vi "main.vi"(11 "VI Refnum":refnum<vi>) -> ()   [LabVIEW 2013]
panel:
  out "Array":string[](array[string])
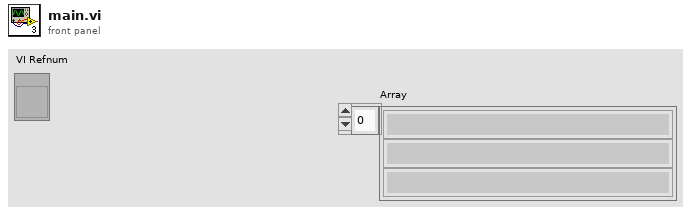
[diagram p1: front panel]
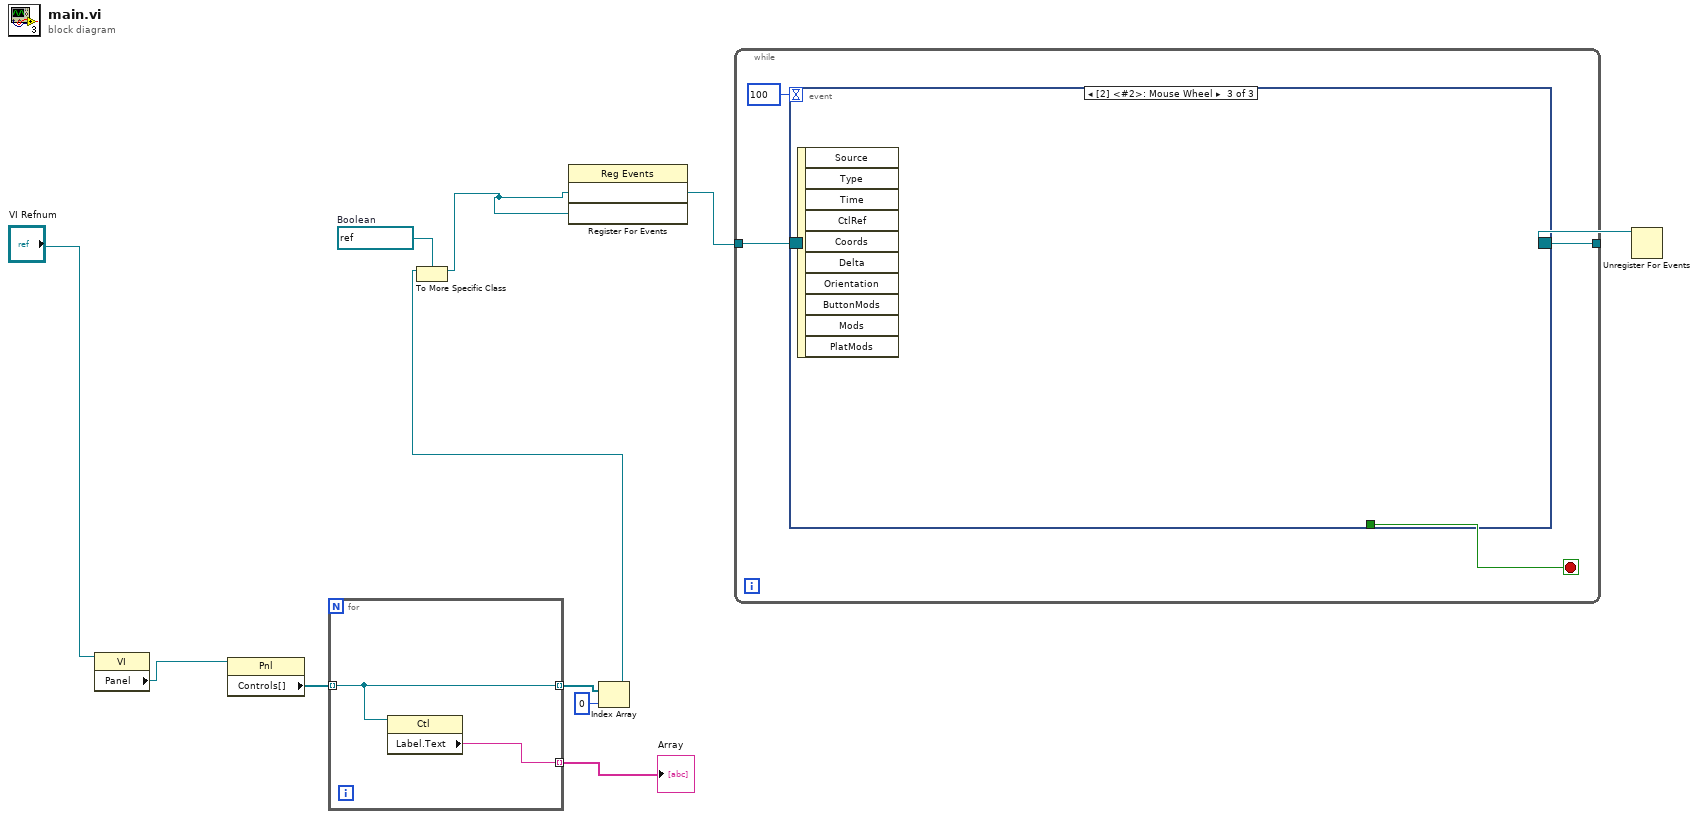
[diagram p0: block diagram]
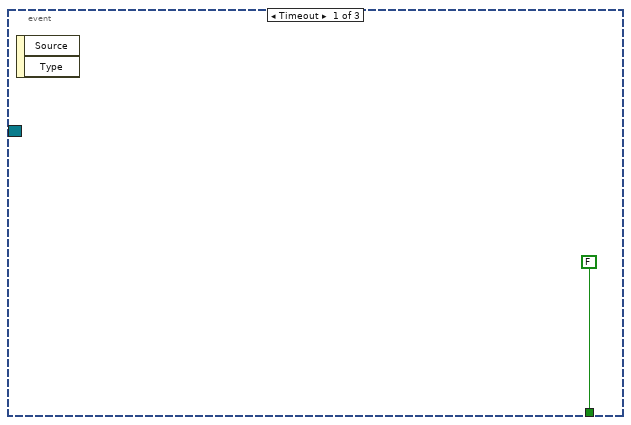
[diagram p2: hidden frame]
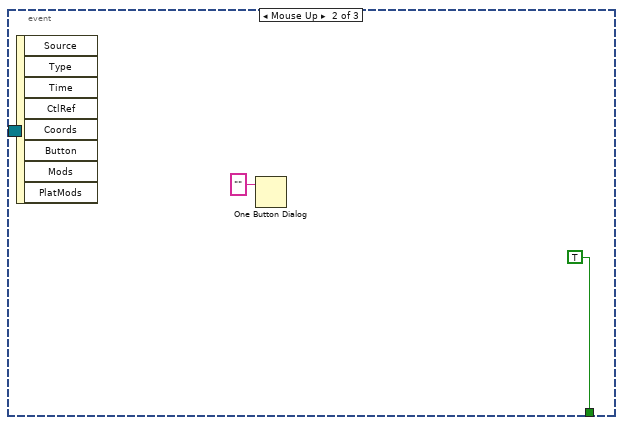
[diagram p3: hidden frame]
diagram:
  w2 = refnum<vi> refnum  # Boolean
  n1 = property class="VI"(reference="VI Refnum") -> ("Panel"=w10:refnum<vi>)  [unwired: 1 in, 2 out]
  n2 = property class="Pnl"(reference=w10) -> ("Controls[]"=w9:refnum<vi>[])  [unwired: 1 in, 2 out]
  n3 = for {
    tunnel: w9 -> [w12] mode=indexing
    tunnel: [w13] -> w8 mode=indexing
    tunnel: [w12] -> w6 mode=indexing
    n4 = property class="Ctl"(reference=w12) -> ("Label.Text"=w13:string)  [unwired: 1 in, 2 out]
  }
  "Array" <- w8
  n5 = Index Array(array=w6, index=0) -> (element=w1:refnum<vi>)
  n6 = To More Specific Class(target class=w2, reference=w1) -> (specific class reference=w3:refnum<vi>)  [unwired: 1 in, 1 out]
  n7 = register-events(w3, w3) -> (reference out=w4:refnum<event-registration>)  [unwired: 2 in, 1 out]
  n8 = while {
    tunnel: [w16] -> w7
    tunnel: w4 -> [w14]
    stop <- w17 stop-if-true
    n9 = event shown="[2] <#2>: Mouse Wheel" {
      selector: w14 -> [_ _ _]
      dyn-events: [_ _ _] -> w16
      timeout: 100 -> [_ _ _]
      tunnel: [FALSE TRUE _] -> w17
      event Timeout {
        n10 = event-data() -> ()  [unwired: 1 in, 2 out]
      }
      event Mouse Up {
        n11 = event-data() -> ()  [unwired: 1 in, 8 out]
        n12 = One Button Dialog(message="") -> ()  [unwired: 1 in, 1 out]
      }
      event Mouse Wheel {
        n13 = event-data() -> ()  [unwired: 1 in, 10 out]
      }
    }
  }
  n14 = Unregister For Events(event registration refnum=w7) -> ()  [unwired: 1 in, 1 out]
